vi "CAN test do odczytu.vi"() -> ()   [LabVIEW 2014]
doc: "This example demonstrates frame streaming output using an NI-Embedded CAN for RIO interface. \n\nThis example can run against any input example, assuming you have a properly terminated CAN cable connected to two CAN ports."
uses:
  <vilib>/RioEmbeddedCAN/RioEmbeddedCAN.llb/CANFrameControl.ctl
  <vilib>/Platform/TimedLoop/XDataNode/timing_clust.ctl
  <vilib>/Platform/TimedLoop/XDataNode/nitl_modes.ctl
  <vilib>/Platform/TimedLoop/XDataNode/wakeup.ctl
  <vilib>/Platform/TimedLoop/XDataNode/XDataNode.xnode
  <vilib>/Platform/TimedLoop/XDataNode/XDNodeRunTimeDep.lvlib
panel:
  out "value":T1 {"type" items=["CAN Data", "CAN Remote"]; "identifier" format="%.0x"}
  out "length":i32
  in  "stop":bool
  out "ilosc mesagy":dbl
  out "okres":dbl
  in  "udp":bool
  out "value 2":T1[](array[typedef]) {"type" items=["CAN Data", "CAN Remote"]; "identifier" format="%.0x"}
  out "status udp":bool
  out "ile nowych mesagy":dbl
  in  "ramki 2":bool
  out "new data":bool
  in  "CAN frame 2":T1={"identifier"=2, "extended?"=FALSE, "type"=0, "payload"=[1, 2, 3, 4, 5, 6, 7, 8]} {"type" items=["CAN Data", "CAN Remote"]; "identifier" format="%.0x"}
  in  "odczyt":bool=TRUE
  in  "write":bool
  in  "CAN frame":T1={"identifier"=2, "extended?"=FALSE, "type"=0, "payload"=[1, 2, 3, 4, 5, 6, 7, 8]} {"type" items=["CAN Data", "CAN Remote"]; "identifier" format="%.0x"}
  in  "Hexadecimal?":bool
  out "Frames":string[][](table)
  in  "Number of Frames to Display":i32=5
  in  "receive queue size":u32=500
  in  "baud rate":u32=500000
  in  "interface index":u32
  # "Overview: Demonstrates frame streaming output using an NI-Embedded CAN for RIO interface.\nInstructions: Run the VI."
  # "See VI Info <Ctrl+I> for more information on how to use this example"
  # "Interface Configuration"
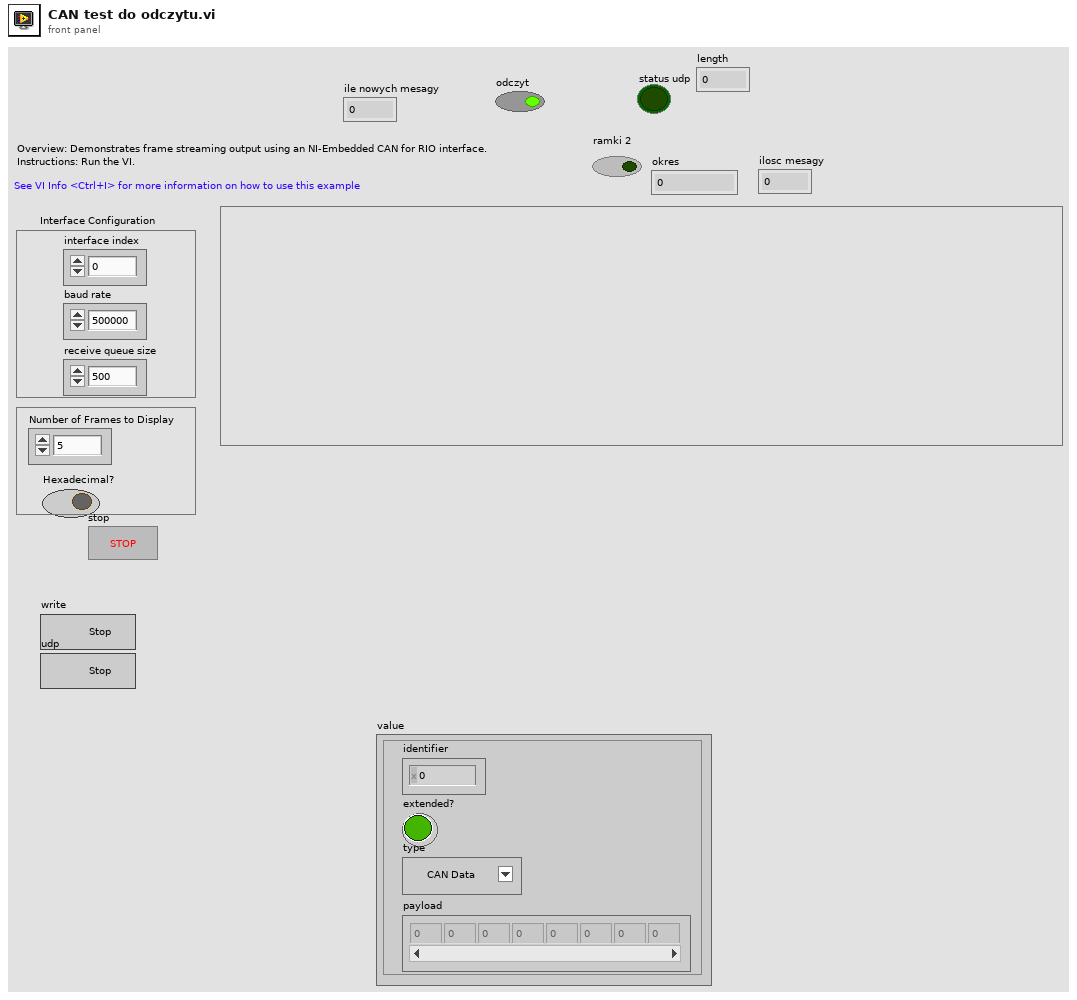
[diagram p1: front panel]
types:
  T1 = typedef "CANFrameControl.ctl" = cluster{"identifier":u32, "extended?":bool, "type":u8, "payload":u8[]}
  T2 = typedef "XDNodeRunTimeDep.lvlib/timing_clust.ctl" = cluster{"Expected End [f-1]":u64, "Actual End [f-1]":u64, "Finished Late? [f-1]":bool, "Expected End [i-1]":u64, "Actual End [i-1]":u64, "Finished Late? [i-1]":bool, "Expected Start [i]":u64, "Actual Start [i]":u64, "Expected Start [f]":u64, "Actual Start [f]":u64, "Source Name":string, "Structure Name":string, "Period":i64, "Deadline":i64, "Offset":i64, "Start":i64, "Priority":i32, "Timeout":i32, "Mode":T3, "Wakeup Reason":T4, "Error":errorcluster, "Source Type":string, "Secondary Source Type":string, "Global End Time":u64, "Global Start Time":u64, "Frame Duration":u64, "Iteration Duration":u64, "Assigned CPU":i32, "I/O Scan Engine Mode":u32}
  T3 = typedef "XDNodeRunTimeDep.lvlib/nitl_modes.ctl" = enum32{"No Change", "Process missed periods, maintain original phase", "Discard missed periods, maintain original phase", "Process missed periods, ignore original phase", "Discard missed periods, ignore original phase"}
  T4 = typedef "XDNodeRunTimeDep.lvlib/wakeup.ctl" = enum32{"Normal", "Aborted", "Asynchronous wakeup", "Timing source error", "Timed loop error", "Timeout"}
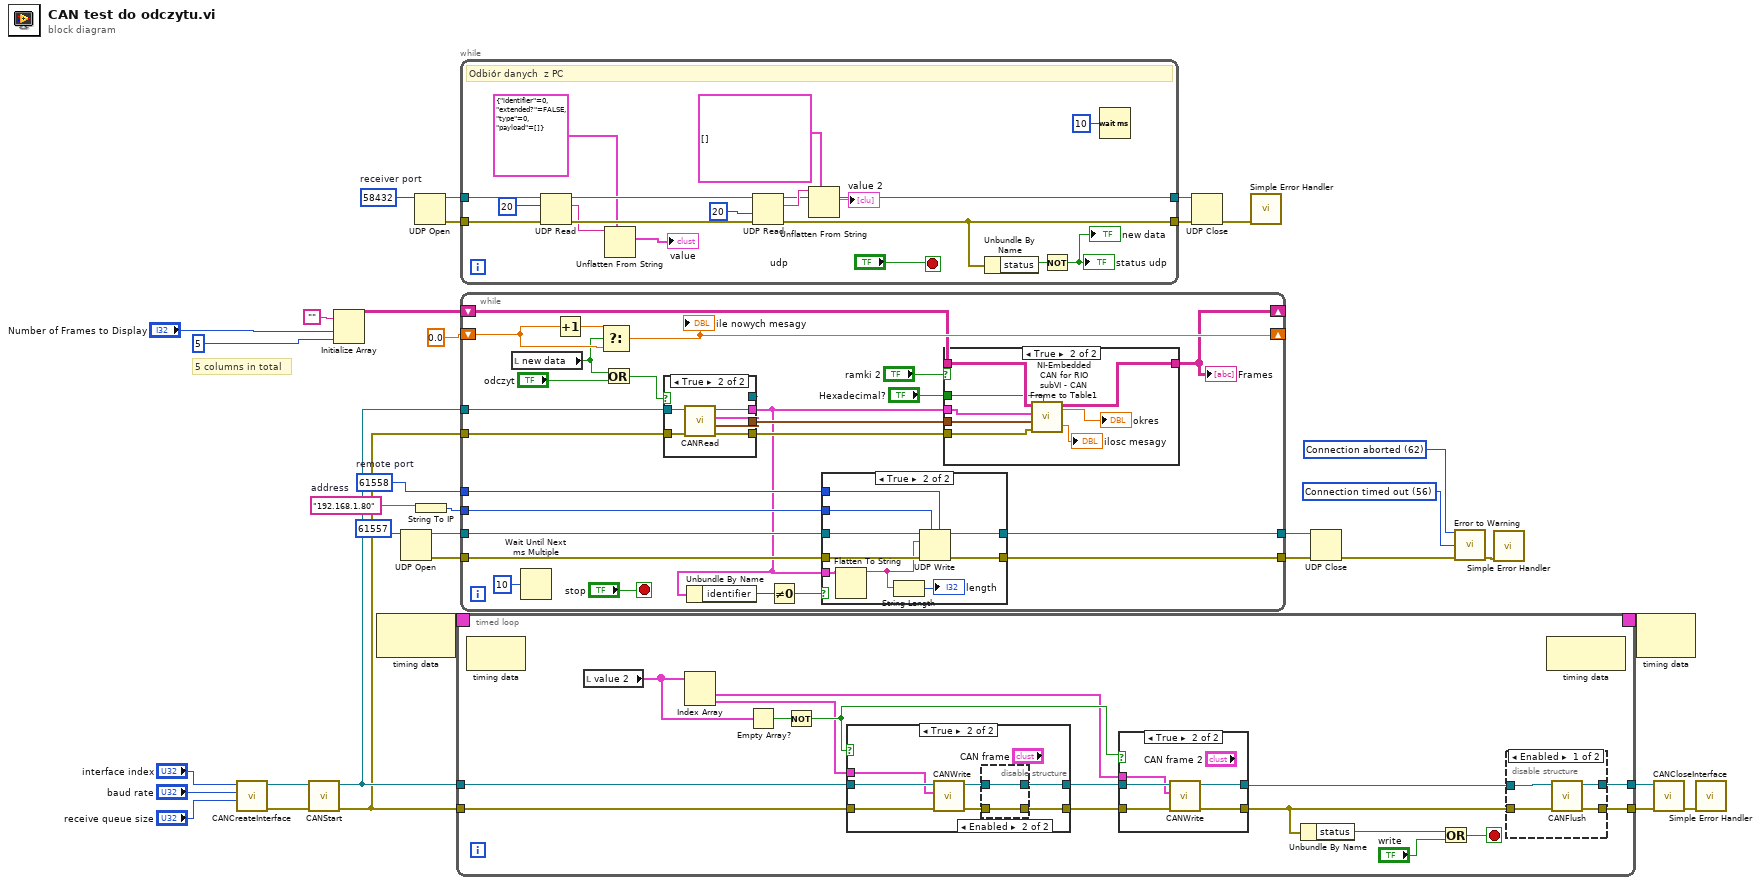
[diagram p0: block diagram]
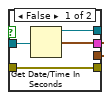
[diagram p4: hidden frame]
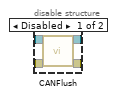
[diagram p8: hidden frame]
diagram:
  w6 = u16 61558  # remote port
  w7 = "192.168.1.80"  # address
  w10 = 56 items=["No Error", "Argument Error", "Memory Full", "Out of Zone", "End of File", "File Already Open", "Generic File IO Error", "File Not Found", "File Permission Error", "Disk Full", "Duplicate Path", "Too Many Files Open", "Not Enabled", "Resource File Not Found", "Cannot Add Resource", "Resource Not Found", "Image Not Found", "Image Memory Error", "Pen Does Not Exist", "Config Bad Type", "Config Token Not Found", "Config Parse Error", "Config Memory Error", "Bad External Code Format", "Bad External Code Offset", "External Code Not Present", "Null Window", "Destroy Window Mixup", "Null Menu", "Print Aborted", "Bad Print Record", "Print Driver Error", "Windows Error During Print", "Memory Error During Print", "Print Dialog Error", "Generic Print Error", "Invalid Device Refnum", "Device Not Found", "Device Parameter Error", "Device Unit Error", "Can't Open Device", "Device Call Aborted", "Generic Error", "Cancelled By User", "Object ID Too Low", "Object ID Too High", "Object Not In Heap", "Unknown Heap", "Bad DefProc ID", "DefProc Not In Table", "Message Out Of Range", "Null Method", "Unknown Message", "Manager Call Not Supported", "Bad address", "Connection In progress", "Connection timed out", "Connection is already in progress", "Network attribute not supported", "Network error", "Address in use", "System out of memory", "Connection aborted", "Connection refused", "Connection is not connected", "Connection is already connected", "Connection closed", "Initialize error (interapplication manager)", "Bad occurrence", "Wait on unbound occurrence handler", "Occurrence queue overflow", "Bad path", "Semaphore not signaled", "Unrecognized type (interapplication manager)"] ("3rd Error to Convert")
  w11 = 62 items=["No Error", "Argument Error", "Memory Full", "Out of Zone", "End of File", "File Already Open", "Generic File IO Error", "File Not Found", "File Permission Error", "Disk Full", "Duplicate Path", "Too Many Files Open", "Not Enabled", "Resource File Not Found", "Cannot Add Resource", "Resource Not Found", "Image Not Found", "Image Memory Error", "Pen Does Not Exist", "Config Bad Type", "Config Token Not Found", "Config Parse Error", "Config Memory Error", "Bad External Code Format", "Bad External Code Offset", "External Code Not Present", "Null Window", "Destroy Window Mixup", "Null Menu", "Print Aborted", "Bad Print Record", "Print Driver Error", "Windows Error During Print", "Memory Error During Print", "Print Dialog Error", "Generic Print Error", "Invalid Device Refnum", "Device Not Found", "Device Parameter Error", "Device Unit Error", "Can't Open Device", "Device Call Aborted", "Generic Error", "Cancelled By User", "Object ID Too Low", "Object ID Too High", "Object Not In Heap", "Unknown Heap", "Bad DefProc ID", "DefProc Not In Table", "Message Out Of Range", "Null Method", "Unknown Message", "Manager Call Not Supported", "Bad address", "Connection In progress", "Connection timed out", "Connection is already in progress", "Network attribute not supported", "Network error", "Address in use", "System out of memory", "Connection aborted", "Connection refused", "Connection is not connected", "Connection is already connected", "Connection closed", "Initialize error (interapplication manager)", "Bad occurrence", "Wait on unbound occurrence handler", "Occurrence queue overflow", "Bad path", "Semaphore not signaled", "Unrecognized type (interapplication manager)"] ("1st Error to Convert")
  w19 = u16 58432  # receiver port
  # "5 columns in total"
  n1 = call <vilib>:"CANCreateInterface.vi"("receive queue size (5)"="receive queue size", "baud rate (125000 bps)"="baud rate", "interface index"="interface index") -> ("error out"=w35:errorcluster, "interface object out"=w25:refnum<k20>)  [unwired: 7 in]
  n2 = call <vilib>:"CANStart.vi"("error in (no error)"=w35, "interface object in"=w25) -> ("error out"=w14:errorcluster, "interface object out"=w15:refnum<k20>)  [unwired: 8 in]
  n3 = Initialize Array("" ("Empty String Constant"), "Number of Frames to Display", 5 ("dimension size")) -> (w16:string[][])
  n4 = node-c288() -> (w18:T2)  [unwired: 1 in]
  n5 = UDP Open(11:u16 61557 ("port")) -> (port=w4:refnum<k16>, 0:w3:errorcluster)  [unwired: 4 in, 1 out]
  n6 = UDP Open(11:w19) -> (port=w21:refnum<k16>, 0:w22:errorcluster)  [unwired: 4 in, 1 out]
  n7 = String To IP(1:w7) -> (0:w5:u32)
  n8 = timed-loop "Timed Loop" {
    tunnel: w15 -> [w36]
    tunnel: w14 -> [w41]
    tunnel: [w48] -> w27
    tunnel: [w47] -> w26
    timing: w18 -> [_]
    timing-out: [_] -> w17
    stop <- w50 stop-if-true
    n9 = node-c288() -> ()  [unwired: 1 in, 1 out]
    n10 = local read "value 2"() -> (w44:T1[])
    n11 = Index Array(array=w44) -> (element #1=w40:T1, element #2=w39:T1)  [unwired: 2 in]
    n12 = Empty Array?(array=w44) -> (empty?=w43:bool)
    n13 = Not(x=w43) -> (.not. x?=w42:bool)
    n14 = case shown="True" w42 {
      tunnel: w36 -> [w67 w75]
      tunnel: w41 -> [w68 w74]
      tunnel: [w67 w69] -> w45
      tunnel: [w68 w70] -> w46
      tunnel: w39 -> [_ w73]
      frame False {
      }
      frame True {
        n15 = call <vilib>:"CANWrite.vi"("error in (no error)"=w74, "CAN frame"=w73, "interface object in"=w75) -> ("error out"=w72:errorcluster, "interface object out"=w71:refnum<k20>)  [unwired: 7 in]
        n16 = disable-structure shown="Enabled" {
          disable-tunnel: w72 -> [w79 w80]
          disable-tunnel: w71 -> [w78 w81]
          disable-tunnel: [w77 w80] -> w70
          disable-tunnel: [w76 w81] -> w69
          frame Disabled {
            n17 = call <vilib>:"CANFlush.vi"("error in (no error)"=w79, "interface object in"=w78) -> ("error out"=w77:errorcluster, "interface object out"=w76:refnum<k20>)  [unwired: 8 in]
          }
          frame Enabled {
          }
        }
      }
    }
    n18 = case shown="True" w42 {
      tunnel: w46 -> [w55 w60]
      tunnel: [w54 w57] -> w37
      tunnel: [w55 w56] -> w38
      tunnel: w45 -> [w54 w59]
      tunnel: w40 -> [_ w58]
      frame False {
      }
      frame True {
        n19 = call <vilib>:"CANWrite.vi"("error in (no error)"=w60, "CAN frame"=w58, "interface object in"=w59) -> ("error out"=w56:errorcluster, "interface object out"=w57:refnum<k20>)  [unwired: 7 in]
      }
    }
    n20 = Unbundle By Name(w38) -> ("status"=w51:bool)
    n21 = Or(x=w51, y="write") -> (x .or. y?=w50:bool)
    n22 = disable-structure shown="Enabled" {
      disable-tunnel: [w64 w65] -> w48
      disable-tunnel: [w63 w66] -> w47
      disable-tunnel: w37 -> [w62 w65]
      disable-tunnel: w38 -> [w61 w66]
      frame Enabled {
        n23 = call <vilib>:"CANFlush.vi"("error in (no error)"=w61, "interface object in"=w62) -> ("error out"=w63:errorcluster, "interface object out"=w64:refnum<k20>)  [unwired: 8 in]
      }
      frame Disabled {
      }
    }
    n24 = node-c288() -> ()  [unwired: 1 in, 1 out]
  }
  n25 = while {
    tunnel: w21 -> [w89]
    tunnel: w22 -> [w88]
    tunnel: [w95] -> w23
    tunnel: [w97] -> w24
    stop <- "udp" stop-if-true
    # "Odbiór danych  z PC"
    n26 = UDP Read(connection ID=w89, max size (548)=20 ("timeout ms (25000)"), 8:w88) -> (data out=w84:string, error out=w86:errorcluster, 3:w87:refnum<k16>)  [unwired: 1 in, 2 out]
    n27 = Unflatten From String(type=T1 {"identifier"=0, "extended?"=FALSE, "type"=0, "payload"=[]} ("element"), binary string=w84) -> (value=→"value":T1)  [unwired: 3 in, 2 out]
    n28 = UDP Read(connection ID=w87, timeout ms (25000)=20, 8:w86) -> (data out=w98:string, error out=w95:errorcluster, 3:w97:refnum<k16>)  [unwired: 3 out]
    n29 = Unflatten From String(type=T1[] [] ("array of cans"), binary string=w98) -> (value=→"value 2":T1[])  [unwired: 3 in, 2 out]
    n30 = Unbundle By Name(w95) -> ("status"=w94:bool)
    n31 = Not(x=w94) -> (.not. x?=→"new data" →"status udp":bool)
    n32 = Wait (ms)(milliseconds to wait=u32 10) -> ()  [unwired: 1 out]
  }
  n33 = while {
    shift-right: [w116] -> _
    shift-left: w16 -> [w115]
    shift-right: [w120] -> _
    shift-left: 0.0 -> [w121]
    tunnel: w15 -> [w124]
    tunnel: w14 -> [w123]
    tunnel: w6 -> [w106]
    tunnel: w5 -> [w105]
    tunnel: w4 -> [w104]
    tunnel: w3 -> [w103]
    tunnel: [w102] -> w2
    tunnel: [w101] -> w1
    stop <- "stop" stop-if-true
    n34 = local read "new data"() -> (w118:bool)
    n35 = Wait Until Next ms Multiple(millisecond multiple=u32 10) -> ()  [unwired: 1 out]
    n36 = Increment(x=w121) -> (x+1=w122:dbl)
    n37 = Select(t=w122, s=w118, f=w121) -> (s? t:f=w120:dbl)
    "ile nowych mesagy" <- w120
    n38 = Or(x=w118, y="odczyt") -> (x .or. y?=w117:bool)
    n39 = case shown="True" w117 {
      tunnel: w124 -> [w146 w153]
      tunnel: w123 -> [w147 w152]
      tunnel: [w145 w151] -> w114
      tunnel: [w147 w150] -> w113
      tunnel: [_ w148] -> w100
      tunnel: [w146 w149] -> _
      frame False {
        n40 = Get Date/Time In Seconds() -> (seconds since 1Jan1904=w145:timestamp)
      }
      frame True {
        n41 = call <vilib>:"CANRead.vi"("error in (no error)"=w152, "interface object in"=w153) -> ("error out"=w150:errorcluster, "timestamp"=w151:timestamp, "CAN frame"=w148:T1, "interface object out"=w149:refnum<k20>)  [unwired: 6 in]
      }
    }
    n42 = Unbundle By Name(w100) -> ("identifier"=w107:u32)
    n43 = Not Equal To 0?(x=w107) -> (x != 0?=w108:bool)
    n44 = case shown="True" w108 {
      tunnel: [w125 w135] -> w102
      tunnel: w105 -> [_ w134]
      tunnel: w106 -> [_ w133]
      tunnel: w104 -> [w125 w132]
      tunnel: w103 -> [w126 w131]
      tunnel: [w126 w130] -> w101
      tunnel: w100 -> [_ w129]
      frame False {
      }
      frame True {
        n45 = Flatten To String(anything=w129) -> (data string=w128:string)  [unwired: 3 in, 2 out]
        n46 = String Length(string=w128) -> (length=→"length":i32)
        n47 = UDP Write(address=w134, port or service name=w133, connection ID=w132, data in=w128, 8:w131) -> (error out=w130:errorcluster, 3:w135:refnum<k16>)  [unwired: 1 in]
      }
    }
    n48 = case shown="True" "ramki 2" {
      tunnel: [w136 w144] -> w116
      tunnel: w115 -> [w136 w141]
      tunnel: w114 -> [_ w140]
      tunnel: w100 -> [_ w139]
      tunnel: w113 -> [_ w138]
      tunnel: "Hexadecimal?" -> [_ w137]
      frame False {
      }
      frame True {
        n49 = call "NI-Embedded CAN for RIO subVI - CAN Frame to Table1.vi"("Hexadecimal?"=w137, "error in (no error)"=w138, "timestamp"=w140, "CAN frame"=w139, "Input Array"=w141) -> ("Output Array"=w144:string[][], "ilosc mesagy"=→"ilosc mesagy":dbl, "okres 100"=→"okres":dbl)  [unwired: 2 in, 2 out]
      }
    }
    "Frames" <- w116
  }
  n50 = UDP Close(connection ID=w24, 8:w23) -> (error out=w20:errorcluster)  [unwired: 1 out]
  n51 = call <vilib>:"Simple Error Handler.vi"("error in (no error)"=w20) -> ()  [unwired: 1 in, 8 out]
  n52 = UDP Close(connection ID=w2, 8:w1) -> (error out=w12:errorcluster)  [unwired: 1 out]
  n53 = call <vilib>:"Error to Warning.vi"("1st Error to Convert"=w11, "3rd Error to Convert"=w10, "error in"=w12) -> ("warning out"=w9:errorcluster)  [unwired: 3 in, 9 out]
  n54 = call <vilib>:"Simple Error Handler.vi"("error in (no error)"=w9) -> ()  [unwired: 1 in, 8 out]
  n55 = node-c288(w17) -> ()  [unwired: 1 out]
  n56 = call <vilib>:"CANCloseInterface.vi"("error in (no error)"=w26, "interface object in"=w27) -> ("error out"=w28:errorcluster)  [unwired: 9 in]
  n57 = call <vilib>:"Simple Error Handler.vi"("error in (no error)"=w28) -> ()  [unwired: 4 in, 5 out]
